vi "GPIB Send.vi"(9 "text":string, 10 "address":i16, 11 "id":i32) -> (1 "text out":string, 3 "function return":u32)   [LabVIEW 2018, in "AndorSDK.lvlib"]
doc: "EXPNETTYPE unsigned int WINAPI GPIBSend(int id, short address, char * text);"
uses:
  AndorSDK.lvlib
  ATMCD32D.dll
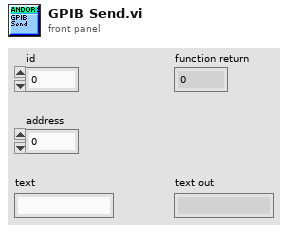
[diagram p1: front panel]
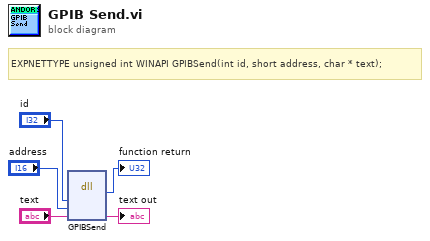
[diagram p0: block diagram]
diagram:
  # "EXPNETTYPE unsigned int WINAPI GPIBSend(int id, short address, char * text);"
  n1 = dll-call lib="PTH2babs E\nPersönliches02 - Arbeit03-HiwijobsLabviewCodelibANDOR\tAndor SDK\nATMCD32D.*" fn="GPIBSend"("id"="id", "address"="address", "text"="text") -> (→"function return":u32, "text"=→"text out":string)  [unwired: 5 in, 2 out]
